vi "Save Header.vi"(8 "error in (no error)":errorcluster, 9 "File Type":string, 10 "Comment String":string, 11 "Configuration Path":path) -> (0 "error out":errorcluster, 1 "Offset for index pointer":i32, 2 "refnum":refnum<file>, 3 "new file path":path, 4 "First section offset":i32)   [LabVIEW 2009]
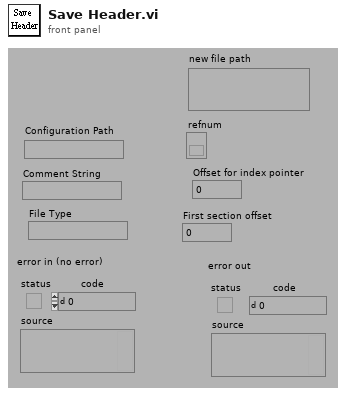
[diagram p1: front panel]
types:
  T1 = enum16{"open", "open or create", "create or replace", "create"}
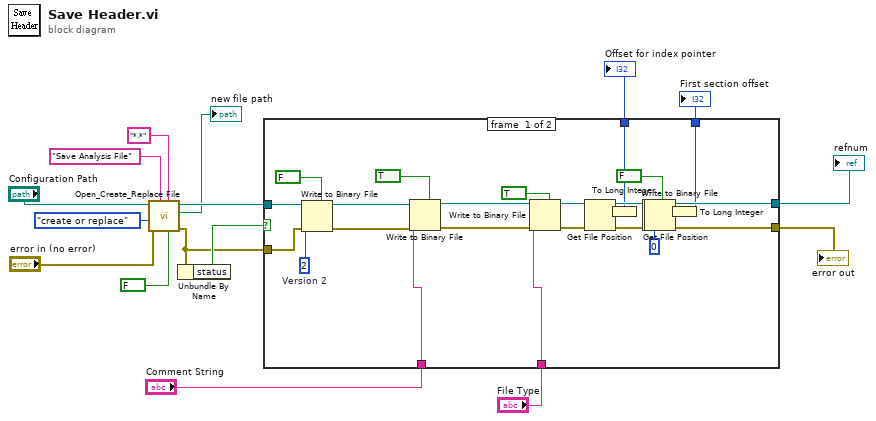
[diagram p0: block diagram]
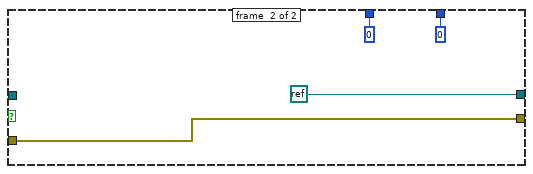
[diagram p2: hidden frame]
diagram:
  n1 = call <vilib>:"Open_Create_Replace File.vi"("advisory dialog? (display:T)"=FALSE, "pattern"="*.*", "prompt"="Save Analysis File", "error in (no error)"="error in (no error)", "function (open:0)"=T1."create or replace", "file path"="Configuration Path") -> ("error out"=w12:errorcluster, "new file path"=→"new file path":path, "refnum"=w11:refnum<file>)  [unwired: 2 in, 1 out]
  n2 = Unbundle By Name(w12) -> ("status"=w13:bool)
  n3 = case shown="False" w13 {
    tunnel: w12 -> [w40 w46]
    tunnel: w11 -> [w41 _]
    tunnel: "Comment String" -> [w37 _]
    tunnel: [w26 refnum<k0> refnum] -> w7
    tunnel: [w25 w46] -> w6
    tunnel: "File Type" -> [w27 _]
    tunnel: [w24 0 ("offset")] -> w2
    tunnel: [w23 0 ("offset")] -> w1
    frame #0 {
      w42 = 2  # Version 2
      n4 = Write to Binary File(file (use dialog)=w41, data=w42, error in=w40, 5:FALSE ("prepend array or string size? (T)")) -> (refnum out=w39:refnum<file>, error out=w38:errorcluster)  [unwired: 2 in, 1 out]
      n5 = Write to Binary File(file (use dialog)=w39, data=w37, error in=w38, 5:TRUE ("header (F)")) -> (refnum out=w29:refnum<file>, error out=w28:errorcluster)  [unwired: 2 in, 1 out]
      n6 = Write to Binary File(file (use dialog)=w29, data=w27, error in=w28, 5:TRUE ("header (F)")) -> (refnum out=w32:refnum<file>, error out=w33:errorcluster)  [unwired: 2 in, 1 out]
      n7 = Get File Position(4:w33, 7:w32) -> (0:w30:errorcluster, 2:w18:i64, 3:w31:refnum<file>)
      n8 = To Long Integer(number=w18) -> (32bit integer=w24:i32)
      n9 = Write to Binary File(file (use dialog)=w31, data=0 ("Index"), error in=w30, 5:FALSE ("prepend array or string size? (T)")) -> (refnum out=w22:refnum<file>, error out=w21:errorcluster)  [unwired: 2 in, 1 out]
      n10 = Get File Position(4:w21, 7:w22) -> (0:w25:errorcluster, 2:w20:i64, 3:w26:refnum<file>)
      n11 = To Long Integer(number=w20) -> (32bit integer=w23:i32)
    }
    frame #1 {
    }
  }
  "error out" <- w6
  "refnum" <- w7
  "Offset for index pointer" <- w2
  "First section offset" <- w1
